vi "Joystick_Control_r2.vi"() -> ()   [LabVIEW 2015]
uses:
  <vilib>/Utility/inputDevices.llb/joystickAcquire.vi
  <vilib>/Utility/inputDevices.llb/closeJoystick.vi
panel:
  in  "Start X":dbl
  in  "Start Y":dbl
  in  "Dest X":dbl
  in  "Dest Y":dbl
  out "Left Duty Cycle 2":dbl=0.5
  out "Right Duty Cycle 2":dbl=0.5
  in  "unjam":bool
  out "Orientation complete":bool
  out "Winch going down":bool
  out "Full":bool
  out "Reverse Diff":dbl
  out "Forward Diff":dbl
  out "Scoop Position":dbl=0.9838866180000001
  out "Drum Accel x":dbl
  out "Winch Accel x":dbl
  in  "Scoops":dbl(knob)=0.075 min=0.05 max=0.1 step=0.005 scale=0.05..0.1
  in  "Winch":dbl(knob)=0.075 min=0.05 max=0.1 step=0.005 scale=0.05..0.1
  in  "Drum":dbl(knob)=0.075 min=0.05 max=0.1 step=0.005 scale=0.05..0.1
  in  "Disable Winch Auto Level":bool
  in  "Disable Drum Auto Level":bool
  out "Current Template - Right":T1(ring)=enum."Range 2"
  out "Current Template - Left":T1(ring)=enum."Range 2"
  in  "Dead wheel speed":dbl(slide)=0.03 min=0.0 max=0.1666 step=0.01 scale=0.0..0.1666
  in  "Stop":bool
  in  "Manual control":bool
  in  "Dump or Mine":dbl(knob) min=-1.0 max=1.0 step=1.0 scale=-1.0..1.0
  in  "stop 2":bool
  out "loc_theta":dbl
  out "loc_y":dbl
  out "loc_x":dbl
  out "Position_Lock":bool
  out "RIGHT_BEACON_BOOL_array":bool[](array[boolean])
  out "LEFT_BEACON_BOOL_array":bool[](array[boolean])
  in  "Start Run":bool
  in  "Auto/Manual":bool
  out "Reverse DC":dbl=0.5
  out "Forward DC":dbl=0.5
  out "Ratio Forward":dbl
  out "Reverse":bool
  out "Right Duty Cycle":dbl=0.5
  out "Left Duty Cycle":dbl=0.5
  out "Right Turn":bool
  out "Left Turn":bool
  in  "stop":bool
  out "Y axis":i32
  out "X axis":i32
  # "1 is the dumping position"
  # "Auto = true\nMaunal = false"
  # "zero is level"
  # "Reverse"
  # "Forward"
  # "Up"
  # "Down"
  # "CW"
  # "CCW"
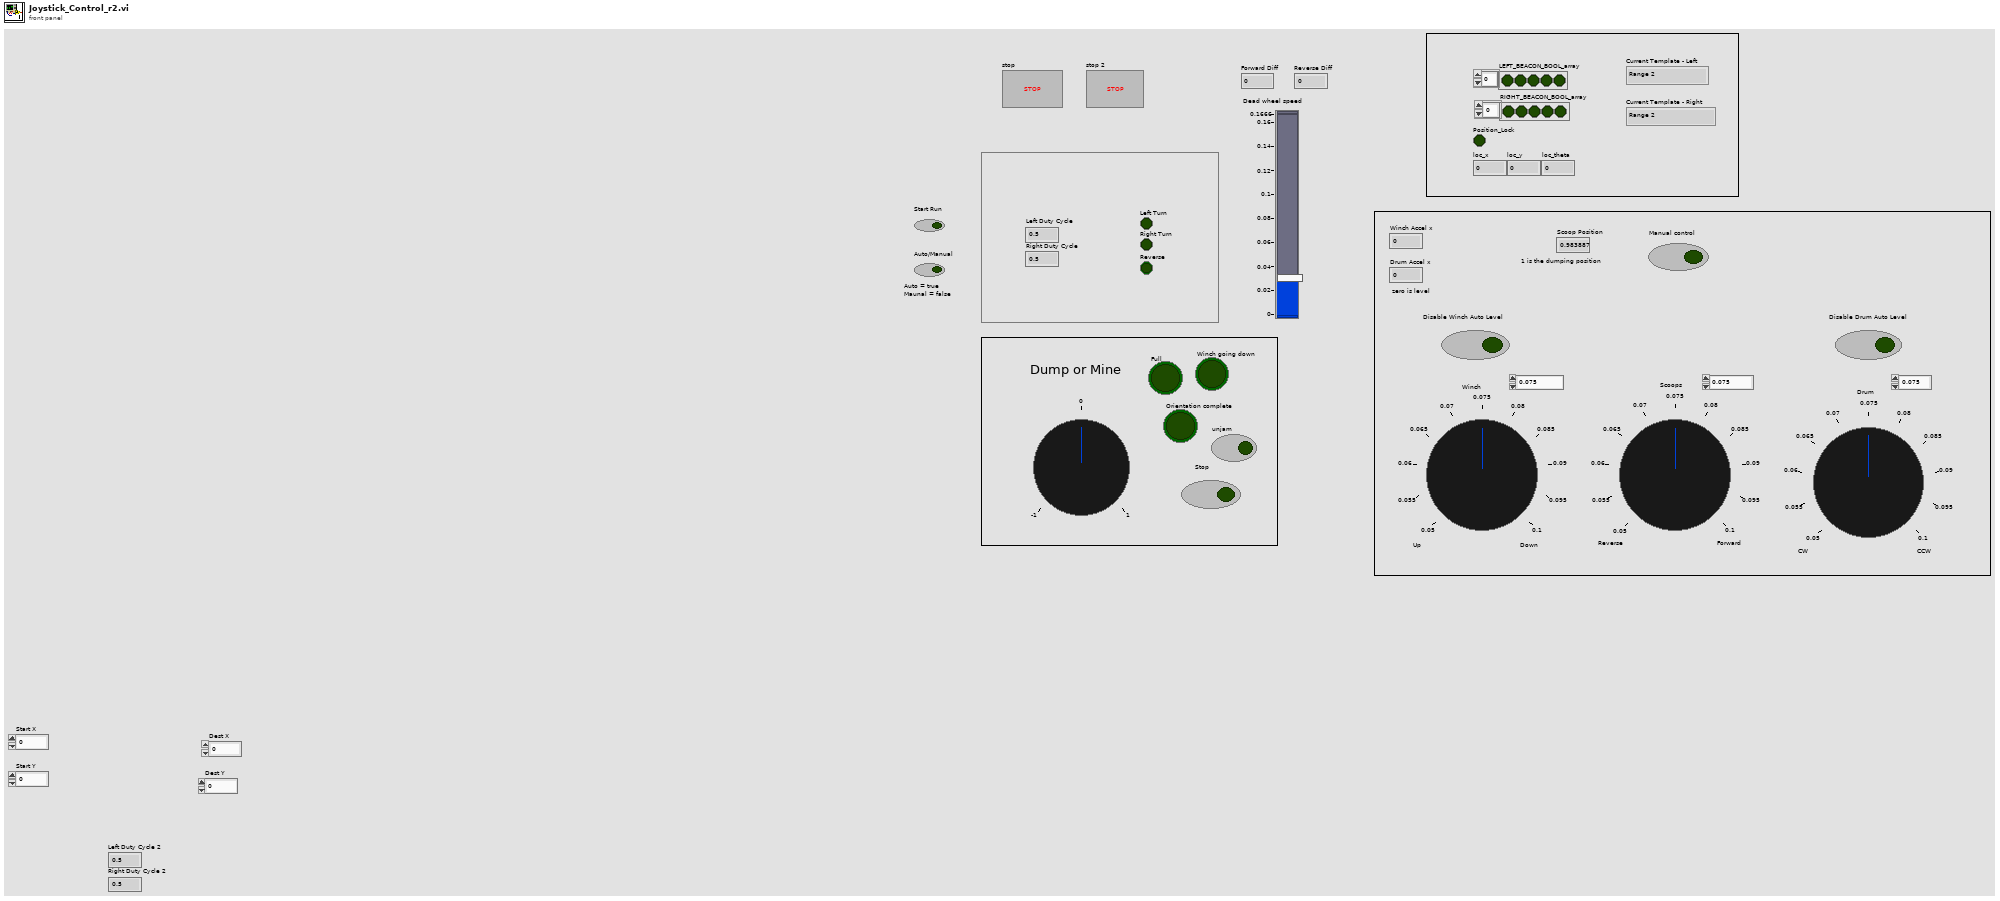
[diagram p1: front panel]
types:
  T1 = enum16{"Range 1", "Range 2", "Range 3", "Range 0"}
  T2 = cluster{"Lock":bool, "Current Valid":bool, "Current Template":enum16{"Range 1", "Range 2", "Range 3", "Range 0"}, "Tracking Coordinates":cluster{"X":dbl, "Y":dbl}, "Setting Values":cluster{"Min Score":dbl, "Min Scale":dbl, "Max Scale":dbl, "Curve Parameters":cluster{"Min Length":i32, "Row Search Step":i32, "Col Search Step":i32}}}
  T3 = cluster{"X axis":i32, "Y axis":i32, "Z axis":i32, "X axis rotation":i32, "Y axis rotation":i32, "Z axis rotation":i32, "U axis":i32, "V axis":i32}
  T4 = cluster{"button 1":bool, "button 2":bool, "button 3":bool, "button 4":bool, "button 5":bool, "button 6":bool, "button 7":bool, "button 8":bool, "button 9":bool, "button 10":bool, "button 11":bool, "button 12":bool, "button 13":bool, "button 14":bool, "button 15":bool, "button 16":bool, "button 17":bool, "button 18":bool, "button 19":bool, "button 20":bool, "button 21":bool, "button 22":bool, "button 23":bool, "button 24":bool, "button 25":bool, "button 26":bool, "button 27":bool, "button 28":bool, "button 29":bool, "button 30":bool, "button 31":bool, "button 32":bool}
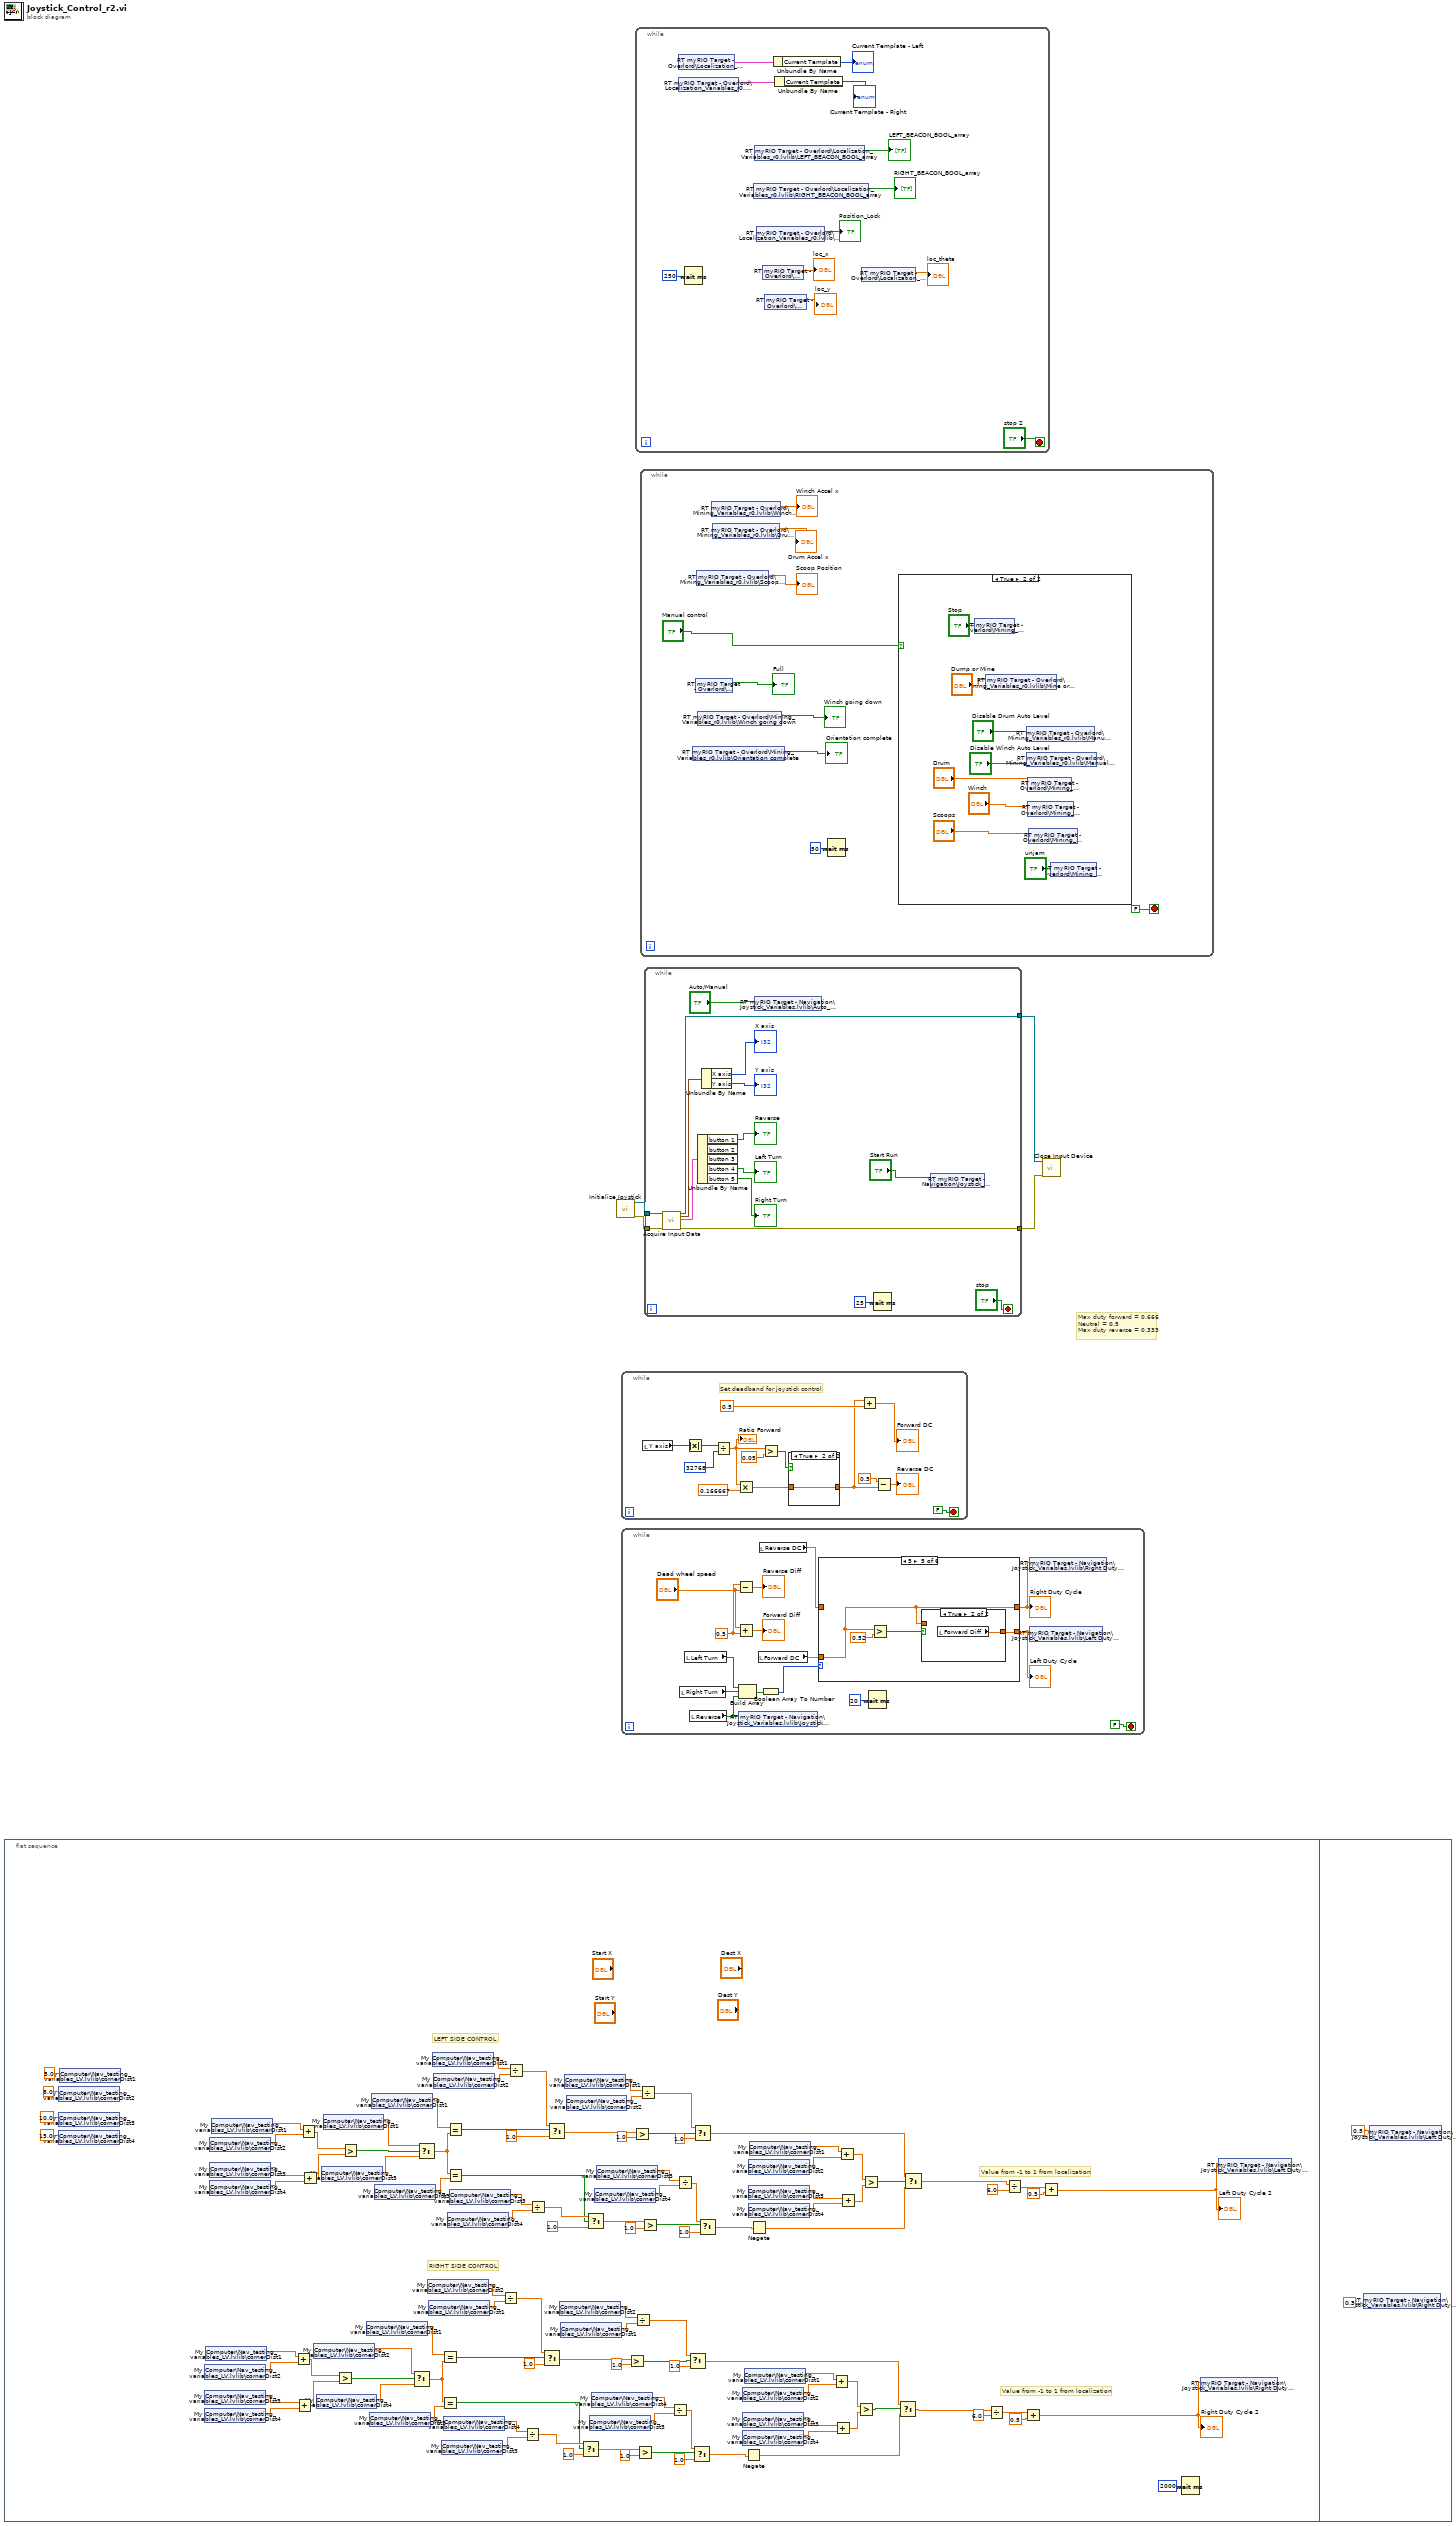
[diagram p0: block diagram]
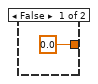
[diagram p3: hidden frame]
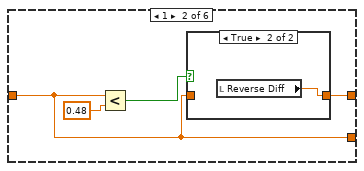
[diagram p5: hidden frame]
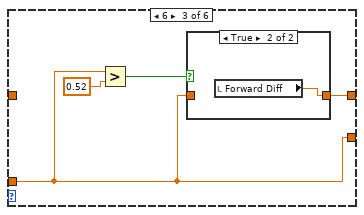
[diagram p7: hidden frame]
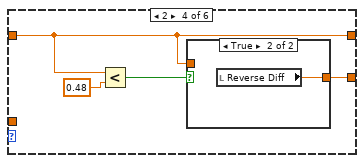
[diagram p9: hidden frame]
diagram:
  # "Max duty forward = 0.666\nNeutral = 0.5\nMax duty reverse = 0.333"
  n1 = flat-sequence {
    frame #0 {
      # "RIGHT SIDE CONTROL"
      # "LEFT SIDE CONTROL"
      # "Value from -1 to 1 from localization"
      # "Value from -1 to 1 from localization"
      n2 = shared-variable "My Computer\\Nav_testing_variables_LV.lvlib\\cornerDist2"(8.0 ("cornerDist2")) -> ()  [unwired: 1 in, 1 out]
      n3 = shared-variable "My Computer\\Nav_testing_variables_LV.lvlib\\cornerDist3"(10.0 ("cornerDist3")) -> ()  [unwired: 1 in, 1 out]
      n4 = shared-variable "My Computer\\Nav_testing_variables_LV.lvlib\\cornerDist4"(15.0 ("cornerDist4")) -> ()  [unwired: 1 in, 1 out]
      n5 = shared-variable "My Computer\\Nav_testing_variables_LV.lvlib\\cornerDist1"(5.0 ("cornerDist1")) -> ()  [unwired: 1 in, 1 out]
      n6 = shared-variable "My Computer\\Nav_testing_variables_LV.lvlib\\cornerDist2"() -> (w52:dbl)  [unwired: 1 in, 1 out]
      n7 = shared-variable "My Computer\\Nav_testing_variables_LV.lvlib\\cornerDist3"() -> (w55:dbl)  [unwired: 1 in, 1 out]
      n8 = shared-variable "My Computer\\Nav_testing_variables_LV.lvlib\\cornerDist4"() -> (w54:dbl)  [unwired: 1 in, 1 out]
      n9 = shared-variable "My Computer\\Nav_testing_variables_LV.lvlib\\cornerDist1"() -> (w53:dbl)  [unwired: 1 in, 1 out]
      n10 = shared-variable "My Computer\\Nav_testing_variables_LV.lvlib\\cornerDist2"() -> (w97:dbl)  [unwired: 1 in, 1 out]
      n11 = shared-variable "My Computer\\Nav_testing_variables_LV.lvlib\\cornerDist3"() -> (w100:dbl)  [unwired: 1 in, 1 out]
      n12 = shared-variable "My Computer\\Nav_testing_variables_LV.lvlib\\cornerDist4"() -> (w99:dbl)  [unwired: 1 in, 1 out]
      n13 = shared-variable "My Computer\\Nav_testing_variables_LV.lvlib\\cornerDist1"() -> (w98:dbl)  [unwired: 1 in, 1 out]
      n14 = Add(x=w53, y=w52) -> (x+y=w58:dbl)
      n15 = Add(x=w55, y=w54) -> (x+y=w57:dbl)
      n16 = Add(x=w98, y=w97) -> (x+y=w103:dbl)
      n17 = Add(x=w100, y=w99) -> (x+y=w102:dbl)
      n18 = shared-variable "My Computer\\Nav_testing_variables_LV.lvlib\\cornerDist2"() -> (w15:dbl)  [unwired: 1 in, 1 out]
      n19 = shared-variable "My Computer\\Nav_testing_variables_LV.lvlib\\cornerDist4"() -> (w51:dbl)  [unwired: 1 in, 1 out]
      n20 = shared-variable "My Computer\\Nav_testing_variables_LV.lvlib\\cornerDist3"() -> (w96:dbl)  [unwired: 1 in, 1 out]
      n21 = shared-variable "My Computer\\Nav_testing_variables_LV.lvlib\\cornerDist1"() -> (w95:dbl)  [unwired: 1 in, 1 out]
      n22 = Greater?(x=w58, y=w57) -> (0:w56:bool)
      n23 = Greater?(x=w103, y=w102) -> (0:w101:bool)
      n24 = shared-variable "My Computer\\Nav_testing_variables_LV.lvlib\\cornerDist1"() -> (w50:dbl)  [unwired: 1 in, 1 out]
      n25 = shared-variable "My Computer\\Nav_testing_variables_LV.lvlib\\cornerDist3"() -> (w48:dbl)  [unwired: 1 in, 1 out]
      n26 = shared-variable "My Computer\\Nav_testing_variables_LV.lvlib\\cornerDist1"() -> (w94:dbl)  [unwired: 1 in, 1 out]
      n27 = shared-variable "My Computer\\Nav_testing_variables_LV.lvlib\\cornerDist3"() -> (w92:dbl)  [unwired: 1 in, 1 out]
      n28 = Select(t=w15, s=w56, f=w51) -> (s? t:f=w49:dbl)
      n29 = Select(t=w95, s=w101, f=w96) -> (s? t:f=w93:dbl)
      n30 = shared-variable "My Computer\\Nav_testing_variables_LV.lvlib\\cornerDist2"() -> (w46:dbl)  [unwired: 1 in, 1 out]
      n31 = shared-variable "My Computer\\Nav_testing_variables_LV.lvlib\\cornerDist1"() -> (w47:dbl)  [unwired: 1 in, 1 out]
      n32 = shared-variable "My Computer\\Nav_testing_variables_LV.lvlib\\cornerDist1"() -> (w90:dbl)  [unwired: 1 in, 1 out]
      n33 = shared-variable "My Computer\\Nav_testing_variables_LV.lvlib\\cornerDist2"() -> (w91:dbl)  [unwired: 1 in, 1 out]
      n34 = Equal?(x=w50, y=w49) -> (x = y?=w45:bool)
      n35 = Equal?(x=w49, y=w48) -> (x = y?=w40:bool)
      n36 = shared-variable "My Computer\\Nav_testing_variables_LV.lvlib\\cornerDist3"() -> (w42:dbl)  [unwired: 1 in, 1 out]
      n37 = shared-variable "My Computer\\Nav_testing_variables_LV.lvlib\\cornerDist4"() -> (w43:dbl)  [unwired: 1 in, 1 out]
      n38 = Equal?(x=w94, y=w93) -> (x = y?=w89:bool)
      n39 = Equal?(x=w93, y=w92) -> (x = y?=w84:bool)
      n40 = shared-variable "My Computer\\Nav_testing_variables_LV.lvlib\\cornerDist4"() -> (w86:dbl)  [unwired: 1 in, 1 out]
      n41 = shared-variable "My Computer\\Nav_testing_variables_LV.lvlib\\cornerDist3"() -> (w87:dbl)  [unwired: 1 in, 1 out]
      n42 = Divide(x=w46, y=w47) -> (x/y=w44:dbl)
      n43 = Divide(x=w90, y=w91) -> (x/y=w88:dbl)
      n44 = Divide(x=w43, y=w42) -> (x/y=w41:dbl)
      n45 = Divide(x=w87, y=w86) -> (x/y=w85:dbl)
      n46 = Select(t=w44, s=w45, f=1.0) -> (s? t:f=w32:dbl)
      n47 = Select(t=w88, s=w89, f=1.0) -> (s? t:f=w76:dbl)
      n48 = shared-variable "My Computer\\Nav_testing_variables_LV.lvlib\\cornerDist2"() -> (w27:dbl)  [unwired: 1 in, 1 out]
      n49 = shared-variable "My Computer\\Nav_testing_variables_LV.lvlib\\cornerDist1"() -> (w28:dbl)  [unwired: 1 in, 1 out]
      n50 = shared-variable "My Computer\\Nav_testing_variables_LV.lvlib\\cornerDist1"() -> (w71:dbl)  [unwired: 1 in, 1 out]
      n51 = shared-variable "My Computer\\Nav_testing_variables_LV.lvlib\\cornerDist2"() -> (w72:dbl)  [unwired: 1 in, 1 out]
      n52 = Select(t=w41, s=w40, f=1.0) -> (s? t:f=w39:dbl)
      n53 = Select(t=w85, s=w84, f=1.0) -> (s? t:f=w83:dbl)
      n54 = shared-variable "My Computer\\Nav_testing_variables_LV.lvlib\\cornerDist3"() -> (w36:dbl)  [unwired: 1 in, 1 out]
      n55 = shared-variable "My Computer\\Nav_testing_variables_LV.lvlib\\cornerDist4"() -> (w37:dbl)  [unwired: 1 in, 1 out]
      n56 = shared-variable "My Computer\\Nav_testing_variables_LV.lvlib\\cornerDist4"() -> (w80:dbl)  [unwired: 1 in, 1 out]
      n57 = shared-variable "My Computer\\Nav_testing_variables_LV.lvlib\\cornerDist3"() -> (w81:dbl)  [unwired: 1 in, 1 out]
      n58 = Greater?(x=w32, y=1.0) -> (0:w30:bool)
      n59 = Greater?(x=w76, y=1.0) -> (0:w74:bool)
      n60 = Divide(x=w27, y=w28) -> (x/y=w26:dbl)
      n61 = Greater?(x=w39, y=1.0) -> (0:w35:bool)
      n62 = Divide(x=w71, y=w72) -> (x/y=w70:dbl)
      n63 = Greater?(x=w83, y=1.0) -> (0:w79:bool)
      n64 = Divide(x=w37, y=w36) -> (x/y=w34:dbl)
      n65 = Divide(x=w81, y=w80) -> (x/y=w78:dbl)
      n66 = Select(t=w26, s=w30, f=1.0) -> (s? t:f=w19:dbl)
      n67 = Select(t=w34, s=w35, f=1.0) -> (s? t:f=w17:dbl)
      n68 = Select(t=w70, s=w74, f=1.0) -> (s? t:f=w63:dbl)
      n69 = Select(t=w78, s=w79, f=1.0) -> (s? t:f=w60:dbl)
      n70 = shared-variable "My Computer\\Nav_testing_variables_LV.lvlib\\cornerDist2"() -> (w22:dbl)  [unwired: 1 in, 1 out]
      n71 = shared-variable "My Computer\\Nav_testing_variables_LV.lvlib\\cornerDist3"() -> (w25:dbl)  [unwired: 1 in, 1 out]
      n72 = shared-variable "My Computer\\Nav_testing_variables_LV.lvlib\\cornerDist4"() -> (w24:dbl)  [unwired: 1 in, 1 out]
      n73 = shared-variable "My Computer\\Nav_testing_variables_LV.lvlib\\cornerDist1"() -> (w23:dbl)  [unwired: 1 in, 1 out]
      n74 = Negate(x=w17) -> (-x=w16:dbl)
      n75 = shared-variable "My Computer\\Nav_testing_variables_LV.lvlib\\cornerDist2"() -> (w66:dbl)  [unwired: 1 in, 1 out]
      n76 = shared-variable "My Computer\\Nav_testing_variables_LV.lvlib\\cornerDist3"() -> (w69:dbl)  [unwired: 1 in, 1 out]
      n77 = shared-variable "My Computer\\Nav_testing_variables_LV.lvlib\\cornerDist4"() -> (w68:dbl)  [unwired: 1 in, 1 out]
      n78 = shared-variable "My Computer\\Nav_testing_variables_LV.lvlib\\cornerDist1"() -> (w67:dbl)  [unwired: 1 in, 1 out]
      n79 = Negate(x=w60) -> (-x=w59:dbl)
      n80 = Add(x=w23, y=w22) -> (x+y=w21:dbl)
      n81 = Add(x=w25, y=w24) -> (x+y=w20:dbl)
      n82 = Add(x=w67, y=w66) -> (x+y=w65:dbl)
      n83 = Add(x=w69, y=w68) -> (x+y=w64:dbl)
      n84 = Greater?(x=w21, y=w20) -> (0:w18:bool)
      n85 = Greater?(x=w65, y=w64) -> (0:w62:bool)
      n86 = Select(t=w19, s=w18, f=w16) -> (s? t:f=w14:dbl)
      n87 = Select(t=w63, s=w62, f=w59) -> (s? t:f=w61:dbl)
      n88 = Divide(x=w14, y=6.0) -> (x/y=w110:dbl)
      n89 = Divide(x=w61, y=6.0) -> (x/y=w106:dbl)
      n90 = Add(x=w110, y=0.5) -> (x+y=w108:dbl)
      "Right Duty Cycle 2" <- w108
      n91 = Add(x=w106, y=0.5) -> (x+y=w104:dbl)
      "Left Duty Cycle 2" <- w104
      n92 = Wait (ms)(milliseconds to wait=u32 2000) -> ()  [unwired: 1 out]
      n93 = shared-variable "RT myRIO Target - Navigation\\Joystick_Variables.lvlib\\Right Duty Cycle"(w108) -> ()  [unwired: 1 in, 1 out]
      n94 = shared-variable "RT myRIO Target - Navigation\\Joystick_Variables.lvlib\\Left Duty Cycle"(w104) -> ()  [unwired: 1 in, 1 out]
    }
    frame #1 {
      n95 = shared-variable "RT myRIO Target - Navigation\\Joystick_Variables.lvlib\\Right Duty Cycle"(0.5 ("Right Duty Cycle 2")) -> ()  [unwired: 1 in, 1 out]
      n96 = shared-variable "RT myRIO Target - Navigation\\Joystick_Variables.lvlib\\Left Duty Cycle"(0.5 ("Left Duty Cycle")) -> ()  [unwired: 1 in, 1 out]
    }
  }
  n97 = call <vilib>:"Initialize Joystick.vi"() -> ("error out"=w2:errorcluster, "device ID"=w4:refnum<k1>)  [unwired: 10 in]
  n98 = while {
    stop <- FALSE stop-if-true
    # "Set deadband for joystick control"
    n99 = local read "Y axis"() -> (w127:i32)
    n100 = Absolute Value(x=w127) -> (abs(x)=w126:i32)
    n101 = Divide(x=w126, y=32768) -> (x/y=w114:dbl)
    "Ratio Forward" <- w114
    n102 = Multiply(x=w114, y=0.166667) -> (x*y=w117:dbl)
    n103 = Greater?(x=w114, y=0.05) -> (0:w115:bool)
    n104 = case shown="True" w115 {
      tunnel: [0.0 ("y") w129] -> w118
      tunnel: w117 -> [_ w129]
      frame False {
      }
      frame True {
      }
    }
    n105 = Add(x=w118, y=0.5) -> (x+y=→"Forward DC":dbl)
    n106 = Subtract(x=0.5, y=w118) -> (x-y=→"Reverse DC":dbl)
  }
  n107 = while {
    stop <- FALSE stop-if-true
    w131 = 0.5
    n108 = local read "Right Turn"() -> (w142:bool)
    n109 = local read "Left Turn"() -> (w143:bool)
    n110 = local read "Reverse"() -> (w134:bool)
    n111 = Subtract(x=w131, y="Dead wheel speed") -> (x-y=→"Reverse Diff":dbl)
    n112 = Add(x="Dead wheel speed", y=w131) -> (x+y=→"Forward Diff":dbl)
    n113 = Build Array(w143, w142, w134) -> (w141:bool[])
    n114 = shared-variable "RT myRIO Target - Navigation\\Joystick_Variables.lvlib\\Joystick Direction"(w134) -> ()  [unwired: 1 in, 1 out]
    n115 = local read "Forward DC"() -> (w137:dbl)
    n116 = local read "Reverse DC"() -> (w136:dbl)
    n117 = Boolean Array To Number(Boolean array=w141) -> (number=w144:u32)
    n118 = case shown="5" w144 {
      tunnel: [w145 w146 w152 w159 w165 w170] -> w138
      tunnel: [w145 w147 w153 w158 w164 w170] -> w139
      tunnel: w137 -> [_ _ w152 _ w164 w170]
      tunnel: w136 -> [w145 w146 _ w158 _ _]
      frame 0, Default {
      }
      frame 1 {
        n119 = Less?(x=w146, y=0.48) -> (x < y?=w149:bool)
        n120 = case shown="True" w149 {
          tunnel: [w150 w151] -> w147
          tunnel: w146 -> [w150 _]
          frame False {
          }
          frame True {
            n121 = local read "Reverse Diff"() -> (w151:dbl)
          }
        }
      }
      frame 6 {
        n122 = Greater?(x=w152, y=0.52) -> (0:w155:bool)
        n123 = case shown="True" w155 {
          tunnel: [w156 w157] -> w153
          tunnel: w152 -> [w156 _]
          frame False {
          }
          frame True {
            n124 = local read "Forward Diff"() -> (w157:dbl)
          }
        }
      }
      frame 2 {
        n125 = Less?(x=w158, y=0.48) -> (x < y?=w160:bool)
        n126 = case shown="True" w160 {
          tunnel: [w162 w163] -> w159
          tunnel: w158 -> [w162 _]
          frame False {
          }
          frame True {
            n127 = local read "Reverse Diff"() -> (w163:dbl)
          }
        }
      }
      frame 5 {
        n128 = Greater?(x=w164, y=0.52) -> (0:w166:bool)
        n129 = case shown="True" w166 {
          tunnel: [w168 w169] -> w165
          tunnel: w164 -> [w168 _]
          frame False {
          }
          frame True {
            n130 = local read "Forward Diff"() -> (w169:dbl)
          }
        }
      }
      frame 4 {
      }
    }
    "Left Duty Cycle" <- w138
    "Right Duty Cycle" <- w139
    n131 = Wait (ms)(milliseconds to wait=u32 20) -> ()  [unwired: 1 out]
    n132 = shared-variable "RT myRIO Target - Navigation\\Joystick_Variables.lvlib\\Right Duty Cycle"(w139) -> ()  [unwired: 1 in, 1 out]
    n133 = shared-variable "RT myRIO Target - Navigation\\Joystick_Variables.lvlib\\Left Duty Cycle"(w138) -> ()  [unwired: 1 in, 1 out]
  }
  n134 = while {
    stop <- "stop 2" stop-if-true
    n135 = shared-variable "RT myRIO Target - Overlord\\Localization_Variables_r0.lvlib\\Info - Right"() -> (w173:T2)  [unwired: 1 in, 1 out]
    n136 = shared-variable "RT myRIO Target - Overlord\\Localization_Variables_r0.lvlib\\Info - Left"() -> (w174:T2)  [unwired: 1 in, 1 out]
    n137 = Wait (ms)(milliseconds to wait=u32 250) -> ()  [unwired: 1 out]
    n138 = shared-variable "RT myRIO Target - Overlord\\Localization_Variables_r0.lvlib\\RIGHT_BEACON_BOOL_array"() -> (→"RIGHT_BEACON_BOOL_array":bool[])  [unwired: 1 in, 1 out]
    n139 = shared-variable "RT myRIO Target - Overlord\\Localization_Variables_r0.lvlib\\LEFT_BEACON_BOOL_array"() -> (→"LEFT_BEACON_BOOL_array":bool[])  [unwired: 1 in, 1 out]
    n140 = shared-variable "RT myRIO Target - Overlord\\Localization_Variables_r0.lvlib\\Position_Lock"() -> (→"Position_Lock":bool)  [unwired: 1 in, 1 out]
    n141 = shared-variable "RT myRIO Target - Overlord\\Localization_Variables_r0.lvlib\\loc_x"() -> (→"loc_x":dbl)  [unwired: 1 in, 1 out]
    n142 = shared-variable "RT myRIO Target - Overlord\\Localization_Variables_r0.lvlib\\loc_y"() -> (→"loc_y":dbl)  [unwired: 1 in, 1 out]
    n143 = Unbundle By Name(w174) -> ("Current Template"=→"Current Template - Left":T1)
    n144 = Unbundle By Name(w173) -> ("Current Template"=→"Current Template - Right":T1)
    n145 = shared-variable "RT myRIO Target - Overlord\\Localization_Variables_r0.lvlib\\loc_theta"() -> (→"loc_theta":dbl)  [unwired: 1 in, 1 out]
  }
  n146 = while {
    stop <- FALSE stop-if-true
    n147 = shared-variable "RT myRIO Target - Overlord\\Mining_Variables_r0.lvlib\\Orientation complete"() -> (→"Orientation complete":bool)  [unwired: 1 in, 1 out]
    n148 = shared-variable "RT myRIO Target - Overlord\\Mining_Variables_r0.lvlib\\Full"() -> (→"Full":bool)  [unwired: 1 in, 1 out]
    n149 = shared-variable "RT myRIO Target - Overlord\\Mining_Variables_r0.lvlib\\Scoop Position"() -> (→"Scoop Position":dbl)  [unwired: 1 in, 1 out]
    n150 = shared-variable "RT myRIO Target - Overlord\\Mining_Variables_r0.lvlib\\Winch going down"() -> (→"Winch going down":bool)  [unwired: 1 in, 1 out]
    n151 = shared-variable "RT myRIO Target - Overlord\\Mining_Variables_r0.lvlib\\Winch Accel x"() -> (→"Winch Accel x":dbl)  [unwired: 1 in, 1 out]
    n152 = shared-variable "RT myRIO Target - Overlord\\Mining_Variables_r0.lvlib\\Drum Accel x"() -> (→"Drum Accel x":dbl)  [unwired: 1 in, 1 out]
    n153 = Wait (ms)(milliseconds to wait=u32 50) -> ()  [unwired: 1 out]
    n154 = case shown="True" "Manual control" {
      frame False {
      }
      frame True {
        n155 = shared-variable "RT myRIO Target - Overlord\\Mining_Variables_r0.lvlib\\Stop"("Stop") -> ()  [unwired: 1 in, 1 out]
        n156 = shared-variable "RT myRIO Target - Overlord\\Mining_Variables_r0.lvlib\\Mine or Dump"("Dump or Mine") -> ()  [unwired: 1 in, 1 out]
        n157 = shared-variable "RT myRIO Target - Overlord\\Mining_Variables_r0.lvlib\\Manual Drum"("Disable Drum Auto Level") -> ()  [unwired: 1 in, 1 out]
        n158 = shared-variable "RT myRIO Target - Overlord\\Mining_Variables_r0.lvlib\\Manual Winch"("Disable Winch Auto Level") -> ()  [unwired: 1 in, 1 out]
        n159 = shared-variable "RT myRIO Target - Overlord\\Mining_Variables_r0.lvlib\\Drum"("Drum") -> ()  [unwired: 1 in, 1 out]
        n160 = shared-variable "RT myRIO Target - Overlord\\Mining_Variables_r0.lvlib\\Winch"("Winch") -> ()  [unwired: 1 in, 1 out]
        n161 = shared-variable "RT myRIO Target - Overlord\\Mining_Variables_r0.lvlib\\Scoops"("Scoops") -> ()  [unwired: 1 in, 1 out]
        n162 = shared-variable "RT myRIO Target - Overlord\\Mining_Variables_r0.lvlib\\unjam"("unjam") -> ()  [unwired: 1 in, 1 out]
      }
    }
  }
  n163 = while {
    tunnel: w4 -> [w214]
    tunnel: [w213] -> w3
    tunnel: w2 -> [w212]
    tunnel: [w211] -> w1
    stop <- "stop" stop-if-true
    n164 = call-poly <vilib>:"Acquire Input Data.vi"("device ID"=w214, "error in (no error)"=w212) -> ("device ID"=w213:refnum<k1>, "axis info"=w210:T3, "button info"=w209:T4, "error out"=w211:errorcluster)  [unwired: 13 in, 1 out]
    n165 = Unbundle By Name(w209) -> ("button 1"=→"Reverse":bool, "button 4"=→"Left Turn":bool, "button 5"=→"Right Turn":bool)  [unwired: 2 out]
    n166 = Unbundle By Name(w210) -> ("X axis"=→"X axis":i32, "Y axis"=→"Y axis":i32)
    n167 = shared-variable "RT myRIO Target - Navigation\\Joystick_Variables.lvlib\\Auto_Manual"("Auto/Manual") -> ()  [unwired: 1 in, 1 out]
    n168 = Wait (ms)(milliseconds to wait=u32 25) -> ()  [unwired: 1 out]
    n169 = shared-variable "RT myRIO Target - Navigation\\Joystick_Variables.lvlib\\Start Run"("Start Run") -> ()  [unwired: 1 in, 1 out]
  }
  n170 = call-poly <vilib>:"Close Input Device.vi"("error in (no error)"=w1, "device ID"=w3) -> ()  [unwired: 8 in, 1 out]
